vi "Read configuration.vi"(8 "error in":errorcluster, 11 "BuckBoost editor node in":refnum<class "BuckBoost editor node.lvclass">) -> (0 "error out":errorcluster, 2 "configuration":refnum<class "NISE_CEF_serializable configuration.lvclass">, 3 "BuckBoost editor node out":refnum<class "BuckBoost editor node.lvclass">)   [LabVIEW 2017, in "BuckBoost editor node.lvclass"]
uses:
  BuckBoost editor node.lvclass
  <vilib>/NI/Configuration Framework/serializable configuration/NISE_CEF_serializable configuration.lvclass
  BuckBoost editor node.lvclass/BuckBoost editor node.ctl
  module/configuration/BuckBoost configuration.lvclass
  C:/Program Files (x86)/National Instruments/LabVIEW 2017/vi.lib/NI/Configuration Framework/serializable configuration/NISE_CEF_serializable configuration.lvclass
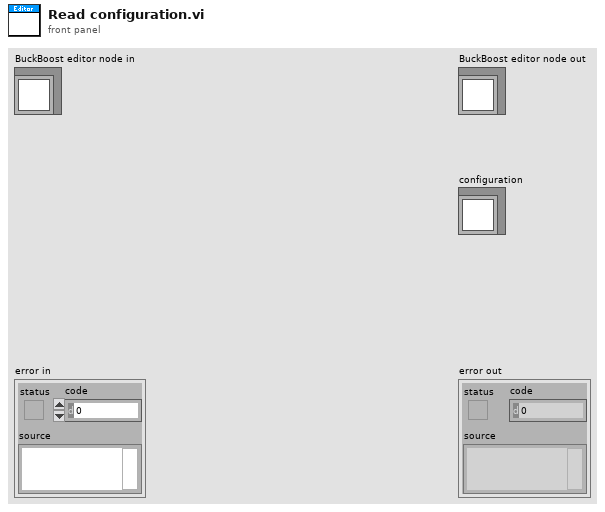
[diagram p1: front panel]
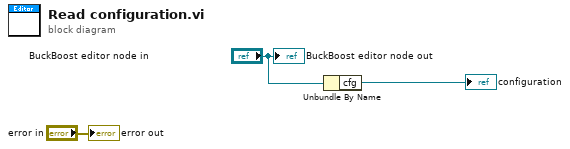
[diagram p0: block diagram]
diagram:
  n1 = Unbundle By Name("BuckBoost editor node in") -> ("cfg"=→"configuration":refnum<class "BuckBoost configuration.lvclass">)
  "error out" <- "error in"
  "BuckBoost editor node out" <- "BuckBoost editor node in"
